vi "Enqueue Multi State.vi"(6 "Priority":T1, 8 "error in (no error)":errorcluster, 10 "Message":T2[](array[typedef]), 11 "QDMH in":refnum<class "QDMH.lvclass">) -> (0 "error out":errorcluster, 3 "QDMH out":refnum<class "QDMH.lvclass">)   [LabVIEW 2023, in "QDMH.lvlib" / "QDMH.lvclass"]
uses:
  QDMH.lvclass
  Custom Controls/QDMH Message.ctl
  Custom Controls/Priority.ctl
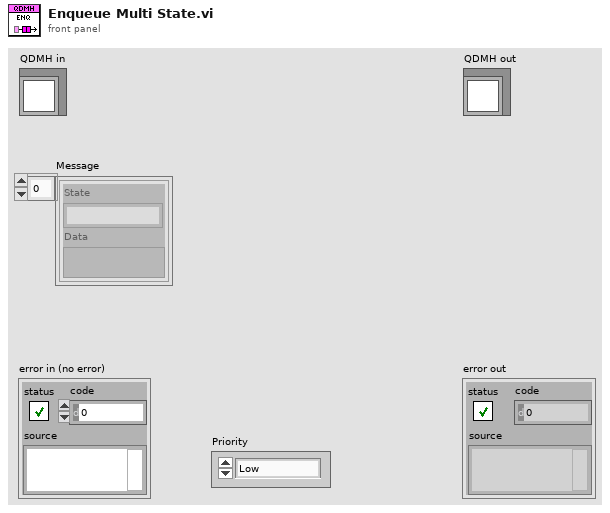
[diagram p1: front panel]
types:
  T1 = typedef "QDMH.lvlib/QDMH.lvclass/Priority.ctl" = enum16{"Low ", "High"}
  T2 = typedef "QDMH.lvlib/QDMH.lvclass/QDMH Message.ctl" = cluster{"State":string, "Data":variant}
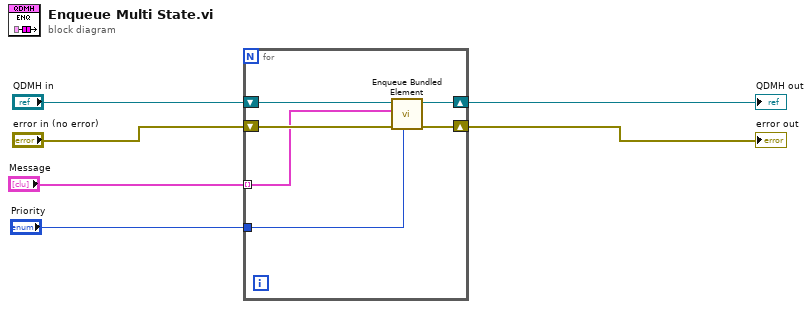
[diagram p0: block diagram]
diagram:
  n1 = for {
    shift-right: [w12] -> w5
    shift-left: "QDMH in" -> [w11]
    shift-right: [w10] -> w3
    shift-left: "error in (no error)" -> [w9]
    tunnel: "Message" -> [w8] mode=indexing
    tunnel: "Priority" -> [w7]
    n2 = call "Enqueue Bundled Element.vi"("Priority(Low)"=w7, "error in"=w9, "element"=w8, "QDMH in"=w11) -> ("error out"=w10:errorcluster, "QDMH out"=w12:refnum<class "QDMH.lvclass">)  [unwired: 6 in]
  }
  "error out" <- w3
  "QDMH out" <- w5
